vi "Write DAT (2D).vi"(4 "Append (0=F)":i32, 6 "Comments":string, 8 "error in":errorcluster, 9 "Data":dbl[][](array[numeric]), 10 "Headers":string[](array[string]), 11 "path":path) -> (0 "error out":errorcluster, 3 "new file path":path)   [LabVIEW 2019, in "Data.DAT.lvclass"]
uses:
  Data.DAT.lvclass
  <vilib>/Utility/file.llb/Write Delimited Spreadsheet (string).vi
  <vilib>/Utility/file.llb/Write Delimited Spreadsheet (DBL).vi
panel:
  out "appended array":string[][](array[string])
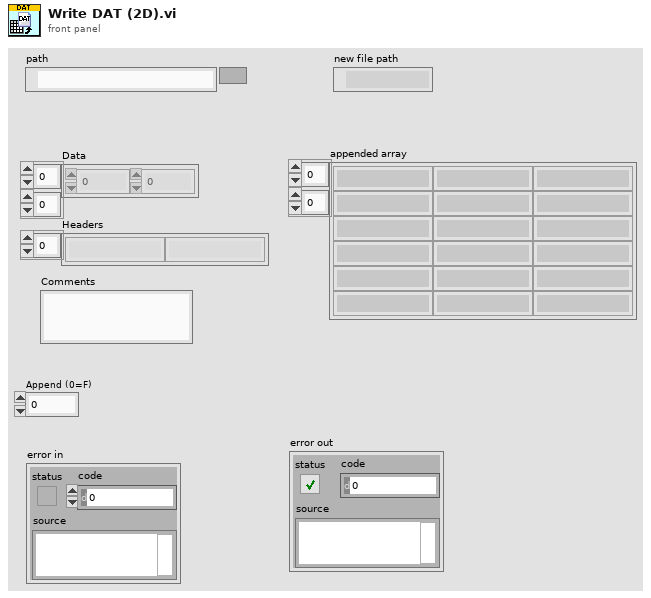
[diagram p1: front panel]
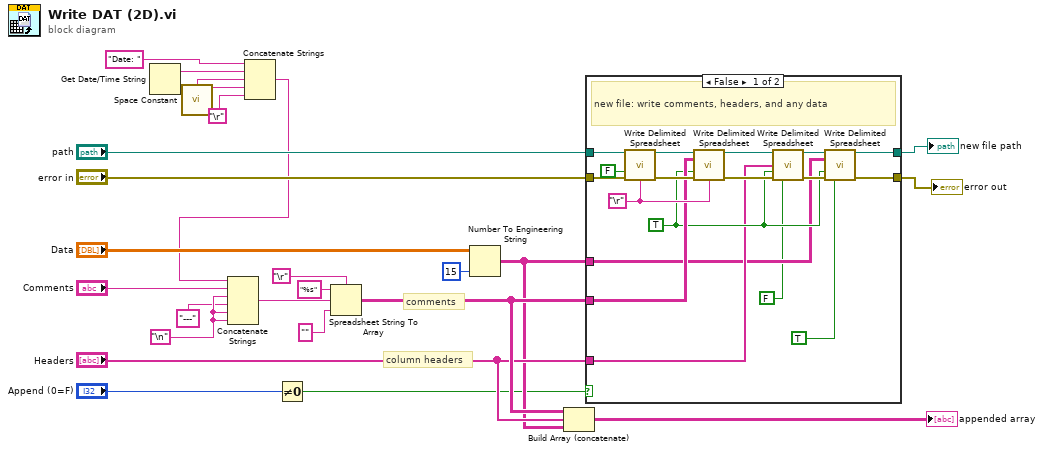
[diagram p0: block diagram]
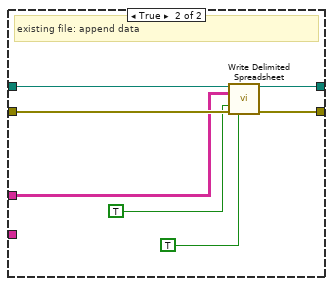
[diagram p2: hidden frame]
diagram:
  w18 = "\n"
  # "comments"
  # "column headers"
  n1 = Get Date/Time String() -> (date string=w6:string, time string=w7:string)  [unwired: 3 out]
  n2 = call <vilib>:"Space Constant.vi"() -> ("String"=w4:string)
  n3 = Concatenate Strings("Date: " ("format string"), w6, w4, w7, "\r") -> (w1:string)
  n4 = Concatenate Strings(w1, "Comments", w18, "---" ("string"), w18, w18) -> (w19:string)
  n5 = Not Equal To 0?(x="Append (0=F)") -> (x != 0?=w8:bool)
  n6 = Spreadsheet String To Array(delimiter (Tab)="\r", format string="%s", spreadsheet string=w19, array type (2D Dbl)="") -> (array=w12:string[][])
  n7 = Number To Engineering String(2:i16 15 ("precision (6)"), 4:"Data") -> (0:w10:string[][])  [unwired: 2 out]
  n8 = Build Array (concatenate)(w12, "Headers", w10) -> (→"appended array":string[][])
  n9 = case shown="False" w8 {
    tunnel: [w37 w48] -> w14
    tunnel: "path" -> [w43 w50]
    tunnel: "error in" -> [w42 w49]
    tunnel: [w38 w47] -> w15
    tunnel: w10 -> [w28 w46]
    tunnel: "Headers" -> [w29 _]
    tunnel: w12 -> [w31 _]
    frame False {
      w30 = TRUE ("append to file? (new file:F)")
      w32 = "\r"
      # "new file: write comments, headers, and any data"
      n10 = call-poly <vilib>:"Write Delimited Spreadsheet.vi"("file path (dialog if empty)"=w43, "append to file? (new file:F)"=FALSE, "error in (no error)"=w42, "delimiter (\\t)"=w32) -> ("new file path (Not A Path if cancelled)"=w35:path, "error out"=w36:errorcluster)  [unwired: 10 in]
      n11 = call-poly <vilib>:"Write Delimited Spreadsheet.vi"("file path (dialog if empty)"=w35, "2D data"=w31, "append to file? (new file:F)"=w30, "error in (no error)"=w36, "delimiter (\\t)"=w32) -> ("new file path (Not A Path if cancelled)"=w34:path, "error out"=w33:errorcluster)  [unwired: 9 in]
      n12 = call-poly <vilib>:"Write Delimited Spreadsheet.vi"("file path (dialog if empty)"=w34, "1D data"=w29, "append to file? (new file:F)"=w30, "error in (no error)"=w33, "transpose? (no:F)"=FALSE) -> ("new file path (Not A Path if cancelled)"=w39:path, "error out"=w40:errorcluster)  [unwired: 9 in]
      n13 = call-poly <vilib>:"Write Delimited Spreadsheet.vi"("file path (dialog if empty)"=w39, "2D data"=w28, "append to file? (new file:F)"=w30, "error in (no error)"=w40, "transpose? (no:F)"=TRUE) -> ("new file path (Not A Path if cancelled)"=w37:path, "error out"=w38:errorcluster)  [unwired: 9 in]
    }
    frame True {
      # "existing file: append data"
      n14 = call-poly <vilib>:"Write Delimited Spreadsheet.vi"("file path (dialog if empty)"=w50, "2D data"=w46, "append to file? (new file:F)"=TRUE, "error in (no error)"=w49, "transpose? (no:F)"=TRUE) -> ("new file path (Not A Path if cancelled)"=w48:path, "error out"=w47:errorcluster)  [unwired: 9 in]
    }
  }
  "new file path" <- w14
  "error out" <- w15
